vi "loop_light_led.vi"(11 "LED":T1) -> ()   [LabVIEW 2016]
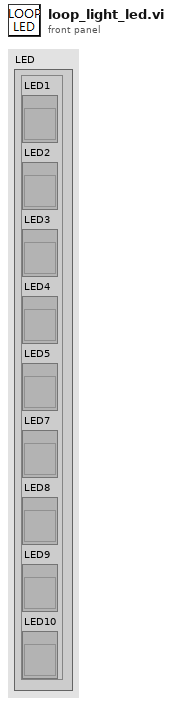
[diagram p1: front panel]
types:
  T1 = cluster{"LED1":refnum<vi>, "LED2":refnum<vi>, "LED3":refnum<vi>, "LED4":refnum<vi>, "LED5":refnum<vi>, "LED7":refnum<vi>, "LED8":refnum<vi>, "LED9":refnum<vi>, "LED10":refnum<vi>}
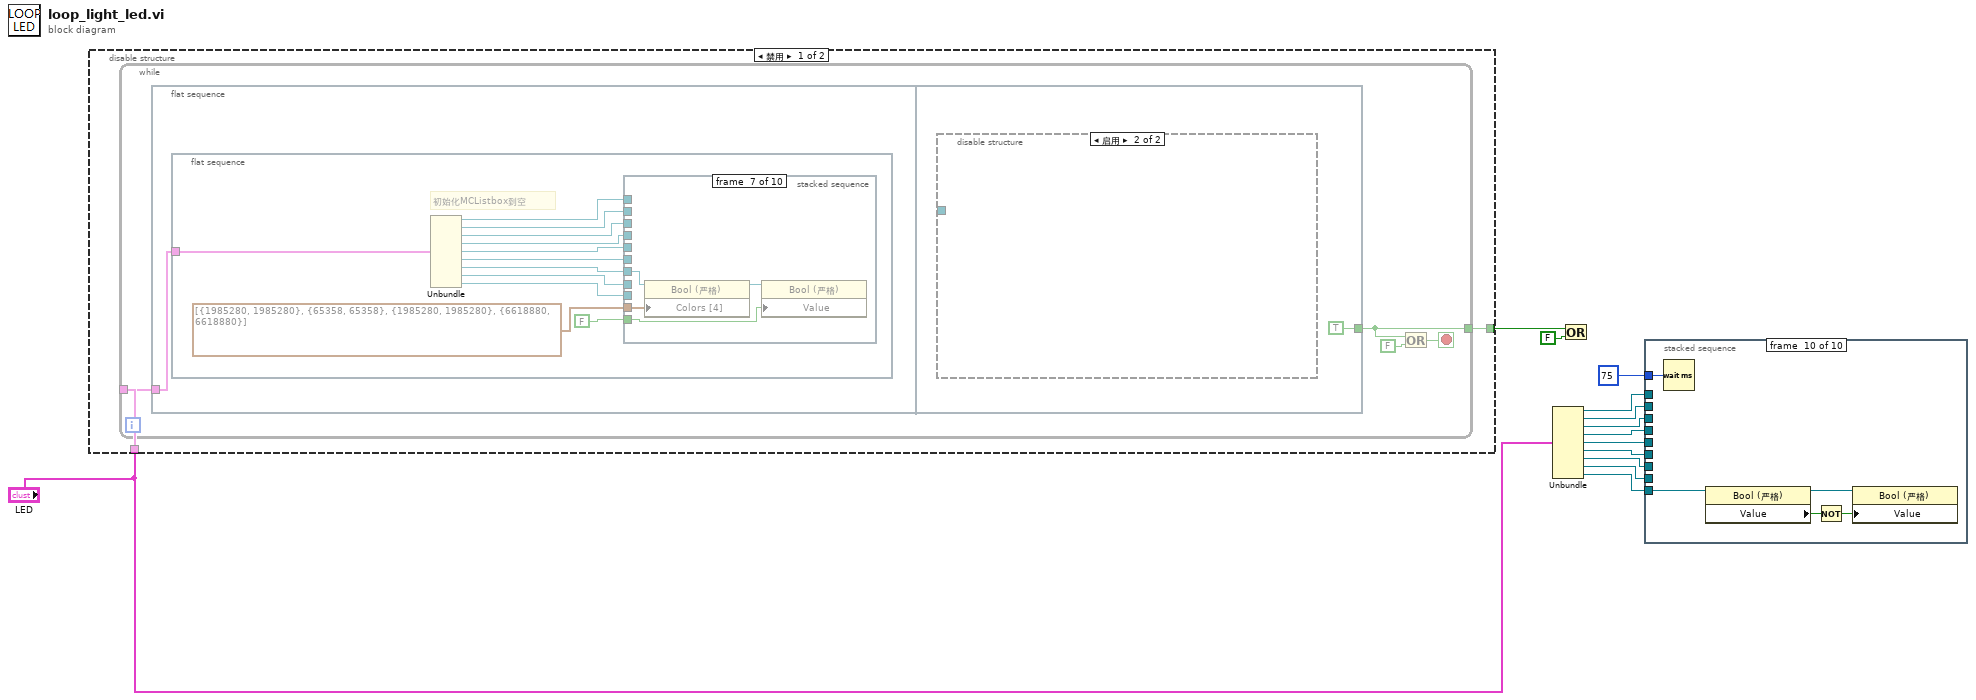
[diagram p0: block diagram]
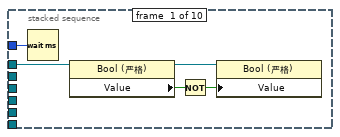
[diagram p2: hidden frame]
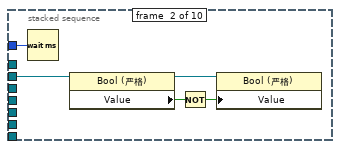
[diagram p3: hidden frame]
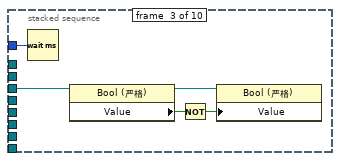
[diagram p4: hidden frame]
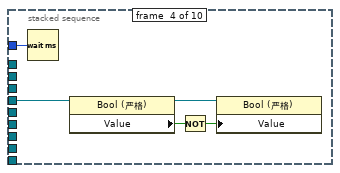
[diagram p5: hidden frame]
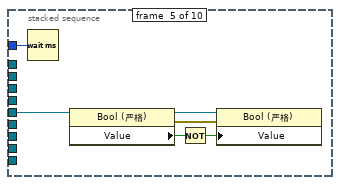
[diagram p6: hidden frame]
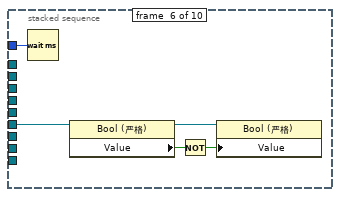
[diagram p7: hidden frame]
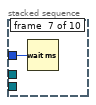
[diagram p8: hidden frame]
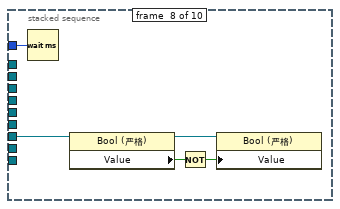
[diagram p9: hidden frame]
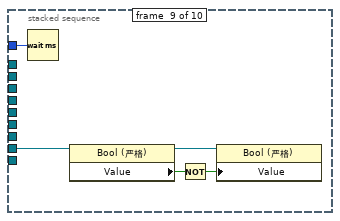
[diagram p10: hidden frame]
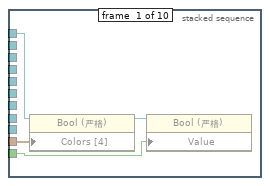
[diagram p11: hidden frame]
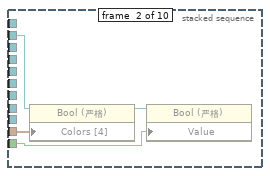
[diagram p12: hidden frame]
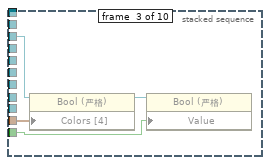
[diagram p13: hidden frame]
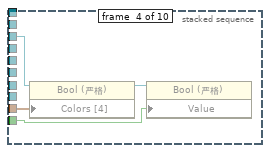
[diagram p14: hidden frame]
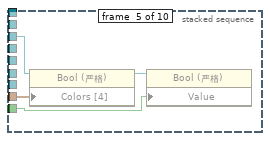
[diagram p15: hidden frame]
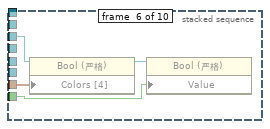
[diagram p16: hidden frame]
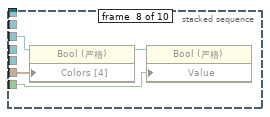
[diagram p17: hidden frame]
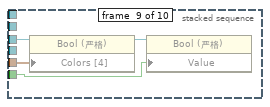
[diagram p18: hidden frame]
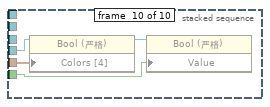
[diagram p19: hidden frame]
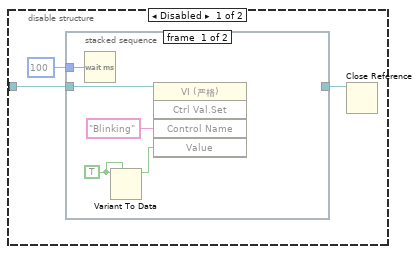
[diagram p20: hidden frame]
diagram:
  n1 = disable-structure shown="禁用" {
    disable-tunnel: [w15 _] -> w13
    disable-tunnel: "LED" -> [w14 _]
    frame Disabled {
      n2 = while {
        tunnel: [w17] -> w15
        tunnel: w14 -> [w16]
        stop <- w18 stop-if-true
        n3 = flat-sequence {
          tunnel: w16 -> [w20]
          tunnel: [TRUE] -> w17
          frame #0 {
            n4 = flat-sequence {
              tunnel: w20 -> [w32]
              frame #0 {
                # "初始化MCListbox到空"
                n5 = Unbundle(w32) -> ("LED1"=w31:refnum<vi>, "LED2"=w30:refnum<vi>, "LED3"=w29:refnum<vi>, "LED4"=w28:refnum<vi>, "LED5"=w27:refnum<vi>, "LED7"=w26:refnum<vi>, "LED8"=w23:refnum<vi>, "LED9"=w24:refnum<vi>, "LED10"=w25:refnum<vi>)
                n6 = stacked-sequence {
                  tunnel: w31 -> [w36 _ _ _ _ _ _ _ _ _]
                  tunnel: w30 -> [_ w40 _ _ _ _ _ _ _ _]
                  tunnel: w29 -> [_ _ w44 _ _ _ _ _ _ _]
                  tunnel: w28 -> [_ _ _ w48 _ _ _ _ _ _]
                  tunnel: w27 -> [_ _ _ _ w52 _ _ _ _ _]
                  tunnel: w26 -> [_ _ _ _ _ w56 _ _ _ _]
                  tunnel: w25 -> [_ _ _ _ _ _ _ _ _ w72]
                  tunnel: w24 -> [_ _ _ _ _ _ _ _ w67 _]
                  tunnel: w23 -> [_ _ _ _ _ _ w60 w64 _ _]
                  tunnel: cluster{u32, u32}[] [{1985280, 1985280}, {65358, 65358}, {1985280, 1985280}, {6618880, 6618880}] ("颜色[4]") -> [w35 w39 w43 w47 w51 w55 w59 w63 w68 w71]
                  tunnel: FALSE -> [w34 w38 w42 w45 w49 w53 w57 w61 w65 w69]
                  frame #0 {
                    n7 = property class="Bool (严格)"(reference=w36, "Colors [4]"=w35) -> (reference out=w33:refnum<vi>)  [unwired: 1 in, 1 out]
                    n8 = property class="Bool (严格)"(reference=w33, "Value"=w34) -> ()  [unwired: 1 in, 2 out]
                  }
                  frame #1 {
                    n9 = property class="Bool (严格)"(reference=w40, "Colors [4]"=w39) -> (reference out=w37:refnum<vi>)  [unwired: 1 in, 1 out]
                    n10 = property class="Bool (严格)"(reference=w37, "Value"=w38) -> ()  [unwired: 1 in, 2 out]
                  }
                  frame #2 {
                    n11 = property class="Bool (严格)"(reference=w44, "Colors [4]"=w43) -> (reference out=w41:refnum<vi>)  [unwired: 1 in, 1 out]
                    n12 = property class="Bool (严格)"(reference=w41, "Value"=w42) -> ()  [unwired: 1 in, 2 out]
                  }
                  frame #3 {
                    n13 = property class="Bool (严格)"(reference=w48, "Colors [4]"=w47) -> (reference out=w46:refnum<vi>)  [unwired: 1 in, 1 out]
                    n14 = property class="Bool (严格)"(reference=w46, "Value"=w45) -> ()  [unwired: 1 in, 2 out]
                  }
                  frame #4 {
                    n15 = property class="Bool (严格)"(reference=w52, "Colors [4]"=w51) -> (reference out=w50:refnum<vi>)  [unwired: 1 in, 1 out]
                    n16 = property class="Bool (严格)"(reference=w50, "Value"=w49) -> ()  [unwired: 1 in, 2 out]
                  }
                  frame #5 {
                    n17 = property class="Bool (严格)"(reference=w56, "Colors [4]"=w55) -> (reference out=w54:refnum<vi>)  [unwired: 1 in, 1 out]
                    n18 = property class="Bool (严格)"(reference=w54, "Value"=w53) -> ()  [unwired: 1 in, 2 out]
                  }
                  frame #6 {
                    n19 = property class="Bool (严格)"(reference=w60, "Colors [4]"=w59) -> (reference out=w58:refnum<vi>)  [unwired: 1 in, 1 out]
                    n20 = property class="Bool (严格)"(reference=w58, "Value"=w57) -> ()  [unwired: 1 in, 2 out]
                  }
                  frame #7 {
                    n21 = property class="Bool (严格)"(reference=w64, "Colors [4]"=w63) -> (reference out=w62:refnum<vi>)  [unwired: 1 in, 1 out]
                    n22 = property class="Bool (严格)"(reference=w62, "Value"=w61) -> ()  [unwired: 1 in, 2 out]
                  }
                  frame #8 {
                    n23 = property class="Bool (严格)"(reference=w67, "Colors [4]"=w68) -> (reference out=w66:refnum<vi>)  [unwired: 1 in, 1 out]
                    n24 = property class="Bool (严格)"(reference=w66, "Value"=w65) -> ()  [unwired: 1 in, 2 out]
                  }
                  frame #9 {
                    n25 = property class="Bool (严格)"(reference=w72, "Colors [4]"=w71) -> (reference out=w70:refnum<vi>)  [unwired: 1 in, 1 out]
                    n26 = property class="Bool (严格)"(reference=w70, "Value"=w69) -> ()  [unwired: 1 in, 2 out]
                  }
                }
              }
            }
          }
          frame #1 {
            n27 = disable-structure shown="启用" {
              disable-tunnel: _ -> [w74 _]
              frame Disabled {
                n28 = stacked-sequence {
                  tunnel: w74 -> [w80 w86]
                  tunnel: 100 -> [w77 w83]
                  tunnel: [_ w82] -> w75
                  frame #0 {
                    w79 = TRUE
                    n29 = Wait (ms)(milliseconds to wait=w77) -> ()  [unwired: 1 out]
                    n30 = Variant To Data(type=w79, Variant=w79) -> (data=w78:bool)  [unwired: 1 in, 1 out]
                    n31 = invoke class="VI (严格)" method="Ctrl Val.Set"(reference=w80, "Control Name"="Blinking" ("控件名"), "Value"=w78) -> ()  [unwired: 2 in, 5 out]
                  }
                  frame #1 {
                    w85 = FALSE
                    n32 = Wait (ms)(milliseconds to wait=w83) -> ()  [unwired: 1 out]
                    n33 = Variant To Data(type=w85, Variant=w85) -> (data=w84:bool)  [unwired: 1 in, 1 out]
                    n34 = invoke class="VI (严格)" method="Ctrl Val.Set"(reference=w86, "Control Name"="Blinking" ("控件名"), "Value"=w84) -> (reference out=w82:refnum<vi>)  [unwired: 2 in, 4 out]
                  }
                }
                n35 = Close Reference(reference=w75) -> ()  [unwired: 1 in, 1 out]
              }
              frame Enabled {
              }
            }
          }
        }
        n36 = Or(x=w17, y=FALSE) -> (x .or. y?=w18:bool)
      }
    }
    frame Enabled {
    }
  }
  n37 = Unbundle("LED") -> ("LED1"=w11:refnum<vi>, "LED2"=w9:refnum<vi>, "LED3"=w8:refnum<vi>, "LED4"=w7:refnum<vi>, "LED5"=w6:refnum<vi>, "LED7"=w5:refnum<vi>, "LED8"=w2:refnum<vi>, "LED9"=w3:refnum<vi>, "LED10"=w4:refnum<vi>)
  n38 = Or(x=w13, y=FALSE) -> ()  [unwired: 1 out]
  n39 = stacked-sequence {
    tunnel: w11 -> [w92 _ _ _ _ _ _ _ _ _]
    tunnel: 75 -> [w88 w95 w98 w103 w109 w116 w119 w122 w125 w132]
    tunnel: w9 -> [_ w97 _ _ _ _ _ _ _ _]
    tunnel: w8 -> [_ _ w99 _ _ _ _ _ _ _]
    tunnel: w7 -> [_ _ _ w107 _ _ _ _ _ _]
    tunnel: w6 -> [_ _ _ _ w108 _ _ _ _ _]
    tunnel: w5 -> [_ _ _ _ _ w115 _ _ _ _]
    tunnel: w4 -> [_ _ _ _ _ _ _ _ _ w134]
    tunnel: w3 -> [_ _ _ _ _ _ _ _ w129 _]
    tunnel: w2 -> [_ _ _ _ _ _ _ w124 _ _]
    frame #0 {
      n40 = Wait (ms)(milliseconds to wait=w88) -> ()  [unwired: 1 out]
      n41 = property class="Bool (严格)"(reference=w92) -> (reference out=w91:refnum<vi>, "Value"=w90:bool)  [unwired: 1 in, 1 out]
      n42 = Not(x=w90) -> (.not. x?=w89:bool)
      n43 = property class="Bool (严格)"(reference=w91, "Value"=w89) -> ()  [unwired: 1 in, 2 out]
    }
    frame #1 {
      n44 = Wait (ms)(milliseconds to wait=w95) -> ()  [unwired: 1 out]
      n45 = property class="Bool (严格)"(reference=w97) -> (reference out=w96:refnum<vi>, "Value"=w94:bool)  [unwired: 1 in, 1 out]
      n46 = Not(x=w94) -> (.not. x?=w93:bool)
      n47 = property class="Bool (严格)"(reference=w96, "Value"=w93) -> ()  [unwired: 1 in, 2 out]
    }
    frame #2 {
      n48 = Wait (ms)(milliseconds to wait=w98) -> ()  [unwired: 1 out]
      n49 = property class="Bool (严格)"(reference=w99) -> (reference out=w100:refnum<vi>, "Value"=w102:bool)  [unwired: 1 in, 1 out]
      n50 = Not(x=w102) -> (.not. x?=w101:bool)
      n51 = property class="Bool (严格)"(reference=w100, "Value"=w101) -> ()  [unwired: 1 in, 2 out]
    }
    frame #3 {
      n52 = Wait (ms)(milliseconds to wait=w103) -> ()  [unwired: 1 out]
      n53 = property class="Bool (严格)"(reference=w107) -> (reference out=w106:refnum<vi>, "Value"=w105:bool)  [unwired: 1 in, 1 out]
      n54 = Not(x=w105) -> (.not. x?=w104:bool)
      n55 = property class="Bool (严格)"(reference=w106, "Value"=w104) -> ()  [unwired: 1 in, 2 out]
    }
    frame #4 {
      n56 = Wait (ms)(milliseconds to wait=w109) -> ()  [unwired: 1 out]
      n57 = property class="Bool (严格)"(reference=w108) -> (reference out=w113:refnum<vi>, error out=w112:errorcluster, "Value"=w111:bool)  [unwired: 1 in]
      n58 = Not(x=w111) -> (.not. x?=w110:bool)
      n59 = property class="Bool (严格)"(reference=w113, error in=w112, "Value"=w110) -> ()  [unwired: 2 out]
    }
    frame #5 {
      n60 = Wait (ms)(milliseconds to wait=w116) -> ()  [unwired: 1 out]
      n61 = property class="Bool (严格)"(reference=w115) -> (reference out=w114:refnum<vi>, "Value"=w118:bool)  [unwired: 1 in, 1 out]
      n62 = Not(x=w118) -> (.not. x?=w117:bool)
      n63 = property class="Bool (严格)"(reference=w114, "Value"=w117) -> ()  [unwired: 1 in, 2 out]
    }
    frame #6 {
      n64 = Wait (ms)(milliseconds to wait=w119) -> ()  [unwired: 1 out]
    }
    frame #7 {
      n65 = Wait (ms)(milliseconds to wait=w122) -> ()  [unwired: 1 out]
      n66 = property class="Bool (严格)"(reference=w124) -> (reference out=w123:refnum<vi>, "Value"=w121:bool)  [unwired: 1 in, 1 out]
      n67 = Not(x=w121) -> (.not. x?=w120:bool)
      n68 = property class="Bool (严格)"(reference=w123, "Value"=w120) -> ()  [unwired: 1 in, 2 out]
    }
    frame #8 {
      n69 = Wait (ms)(milliseconds to wait=w125) -> ()  [unwired: 1 out]
      n70 = property class="Bool (严格)"(reference=w129) -> (reference out=w128:refnum<vi>, "Value"=w127:bool)  [unwired: 1 in, 1 out]
      n71 = Not(x=w127) -> (.not. x?=w126:bool)
      n72 = property class="Bool (严格)"(reference=w128, "Value"=w126) -> ()  [unwired: 1 in, 2 out]
    }
    frame #9 {
      n73 = Wait (ms)(milliseconds to wait=w132) -> ()  [unwired: 1 out]
      n74 = property class="Bool (严格)"(reference=w134) -> (reference out=w133:refnum<vi>, "Value"=w131:bool)  [unwired: 1 in, 1 out]
      n75 = Not(x=w131) -> (.not. x?=w130:bool)
      n76 = property class="Bool (严格)"(reference=w133, "Value"=w130) -> ()  [unwired: 1 in, 2 out]
    }
  }
